vi "Queue check.vi"(11 "output cluster":T2) -> (3 "output cluster 2":T1, 6 "# elements in queue":i32)   [LabVIEW 2015]
uses:
  QMH Fundamentals - Message Cluster.ctl
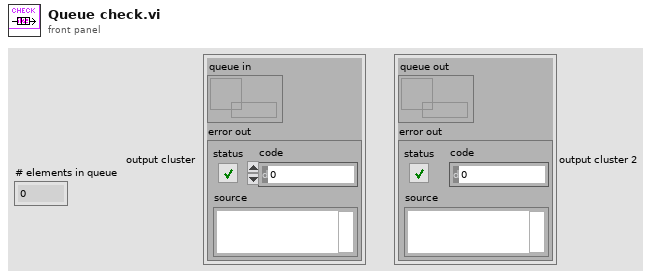
[diagram p1: front panel]
types:
  T1 = cluster{"queue out":refnum<queue>, "error out":errorcluster}
  T2 = cluster{"queue in":refnum<queue>, "error out":errorcluster}
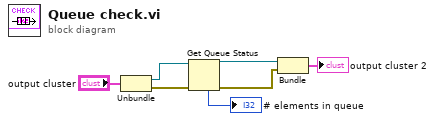
[diagram p0: block diagram]
diagram:
  n1 = Unbundle("output cluster") -> ("queue in"=w6:refnum<queue>, "error out"=w5:errorcluster)
  n2 = Get Queue Status(queue=w6, error in (no error)=w5) -> (queue out=w3:refnum<queue>, error out=w2:errorcluster, # elements in queue=→"# elements in queue":i32)  [unwired: 1 in, 5 out]
  n3 = Bundle("queue in"=w3, "error out"=w2) -> (→"output cluster 2":T2)  [unwired: 1 in]
